vi "Pre-Install Custom Action.vi"(10 "Variant":variant) -> (0 "error out":errorcluster)   [LabVIEW 2020]
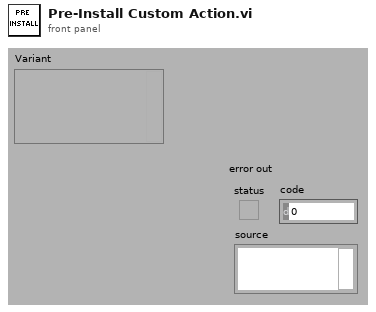
[diagram p1: front panel]
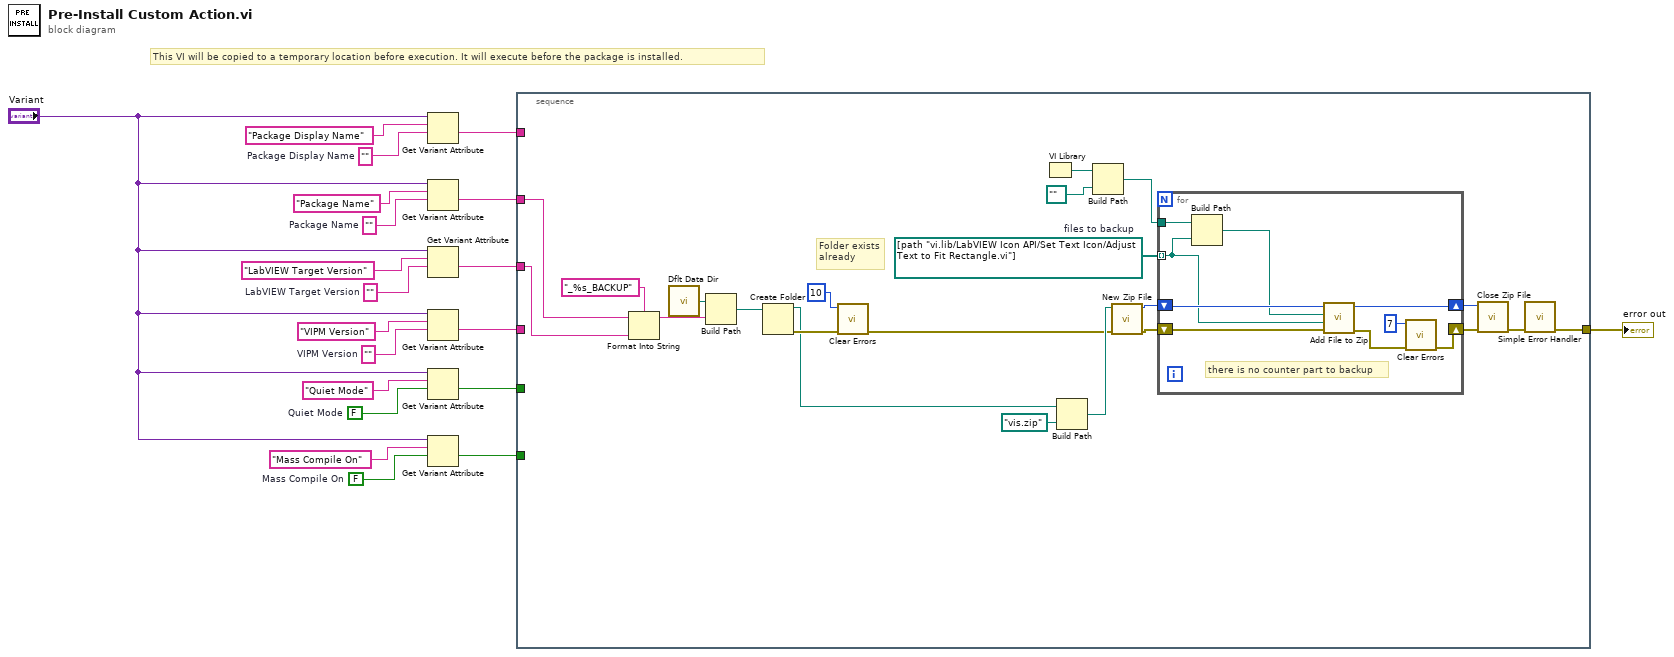
[diagram p0: block diagram]
diagram:
  w2 = FALSE  # Mass Compile On
  w4 = ""  # Package Display Name
  w11 = FALSE  # Quiet Mode
  w14 = ""  # VIPM Version
  w16 = ""  # LabVIEW Target Version
  w18 = ""  # Package Name
  # "This VI will be copied to a temporary location before execution. It will execute before the package is installed."
  n1 = Get Variant Attribute(Variant="Variant", name="Package Display Name", default value (empty Variant)=w4) -> (value=w10:string)  [unwired: 1 in, 3 out]
  n2 = Get Variant Attribute(Variant="Variant", name="Package Name", default value (empty Variant)=w18) -> (value=w9:string)  [unwired: 1 in, 3 out]
  n3 = Get Variant Attribute(Variant="Variant", name="LabVIEW Target Version", default value (empty Variant)=w16) -> (value=w8:string)  [unwired: 1 in, 3 out]
  n4 = Get Variant Attribute(Variant="Variant", name="VIPM Version", default value (empty Variant)=w14) -> (value=w7:string)  [unwired: 1 in, 3 out]
  n5 = Get Variant Attribute(Variant="Variant", name="Quiet Mode", default value (empty Variant)=w11) -> (value=w6:bool)  [unwired: 1 in, 3 out]
  n6 = Get Variant Attribute(Variant="Variant", name="Mass Compile On", default value (empty Variant)=w2) -> (value=w5:bool)  [unwired: 1 in, 3 out]
  n7 = stacked-sequence {
    tunnel: w10 -> [_]
    tunnel: w9 -> [w41]
    tunnel: w8 -> [w40]
    tunnel: w7 -> [_]
    tunnel: w6 -> [_]
    tunnel: w5 -> [_]
    tunnel: [w21] -> w1
    frame #0 {
      w25 = path[] [path "vi.lib/LabVIEW Icon API/Set Text Icon/Adjust Text to Fit Rectangle.vi"]  # files to backup
      # "Folder exists\nalready"
      n8 = Format Into String(format string="_%s_BACKUP", initial string=w41, w40) -> (resulting string=w38:string)  [unwired: 1 in, 1 out]
      n9 = call <vilib>:"Dflt Data Dir.vi"() -> ("App:Default Data Directory"=w39:path)
      n10 = Build Path(base path=w39, name or relative path=w38) -> (appended path=w37:path)
      n11 = Create Folder(path (use dialog)=w37) -> (created path=w23:path, error out=w35:errorcluster)  [unwired: 2 in, 1 out]
      n12 = call <vilib>:"Clear Errors.vi"("error in (no error)"=w35, "specific error code to clear (0: all)"=10) -> ("error out"=w24:errorcluster)  [unwired: 4 in, 1 out]
      n13 = VI Library() -> (path=w30:path)
      n14 = Build Path(base path=w23, name or relative path=path "vis.zip") -> (appended path=w26:path)
      n15 = Build Path(base path=w30, name or relative path=path "..") -> (appended path=w28:path)
      n16 = call <vilib>:"New Zip File.vi"("error in (no error)"=w24, "target"=w26) -> ("error out"=w33:errorcluster, "zip file out"=w34:i64)  [unwired: 3 in, 1 out]
      n17 = for {
        tunnel: w25 -> [w43] mode=indexing
        shift-right: [w46] -> w32
        shift-left: w33 -> [w48]
        shift-right: [w49] -> w31
        shift-left: w34 -> [w50]
        tunnel: w28 -> [w44]
        # "there is no counter part to backup"
        n18 = Build Path(base path=w44, name or relative path=w43) -> (appended path=w47:path)
        n19 = call <vilib>:"Add File to Zip.vi"("error in (no error)"=w48, "destination path in zip"=w43, "source file path"=w47, "zip file in"=w50) -> ("error out"=w51:errorcluster, "zip file out"=w49:i64)  [unwired: 6 in]
        n20 = call <vilib>:"Clear Errors.vi"("error in (no error)"=w51, "specific error code to clear (0: all)"=7) -> ("error out"=w46:errorcluster)  [unwired: 4 in, 1 out]
      }
      n21 = call <vilib>:"Close Zip File.vi"("error in (no error)"=w32, "zip file in"=w31) -> ("error out"=w22:errorcluster)  [unwired: 5 in]
      n22 = call <vilib>:"Simple Error Handler.vi"("error in (no error)"=w22) -> ("error out"=w21:errorcluster)  [unwired: 4 in, 4 out]
    }
  }
  "error out" <- w1
